vi "OpenCSV.vi"(8 "index Delet (row)":i32, 9 "Length Delet":i32=1, 11 "File path":path=path "C:/Users/Notebook/Desktop/OPC Test/Demo_Force_Data.csv") -> (3 "Array Output":T1)   [LabVIEW 2017]
uses:
  <vilib>/Utility/file.llb/Read Delimited Spreadsheet (DBL).vi
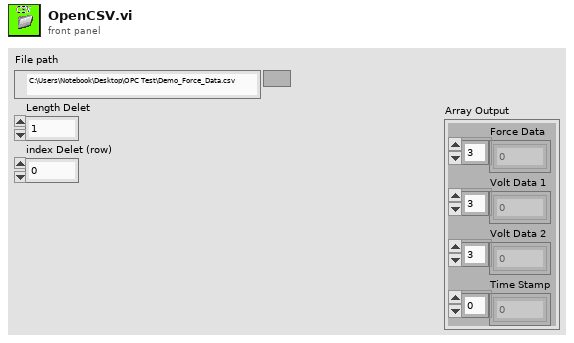
[diagram p1: front panel]
types:
  T1 = cluster{"Force Data":dbl[], "Volt Data 1":dbl[], "Volt Data 2":dbl[], "Time Stamp":dbl[]}
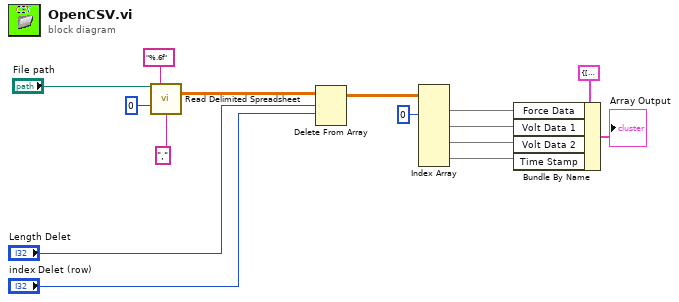
[diagram p0: block diagram]
diagram:
  n1 = call-poly <vilib>:"Read Delimited Spreadsheet.vi"("file path (dialog if empty)"="File path", "format (%.3f)"="%.6f", "max characters/row  (no limit:0)"=0, "delimiter (\\t)"="," ("delimiter (\\t)")) -> ("all rows"=w8:dbl[][])  [unwired: 6 in, 5 out]
  n2 = Delete From Array(array=w8, length="Length Delet", index (row)="index Delet (row)") -> (array with subset deleted=w5:dbl[][])  [unwired: 1 in, 1 out]
  n3 = Index Array(array=w5, index (col) #1=0 ("disabled index (col)")) -> (element #1=w4:dbl[], element #2=w3:dbl[], element #3=w2:dbl[], element #4=w1:dbl[])  [unwired: 7 in]
  n4 = Bundle By Name(cluster=T1 {"Force Data"=[], "Volt Data 1"=[], "Volt Data 2"=[], "Time Stamp"=[]} ("Analog Array In"), "Force Data"=w4, "Volt Data 1"=w3, "Volt Data 2"=w2, "Time Stamp"=w1) -> (→"Array Output":T1)
